vi "TCP Message Loop.vi"(8 "error in (no error)":errorcluster, 10 "Data Notifier":refnum<notifier>, 11 "Message Queues":T1) -> (0 "error out":errorcluster)   [LabVIEW 2026, in "TCP.lvlib"]
uses:
  TCP.lvlib
  Support/Message Queue/All Message Queues.ctl
  Support/Message Queue/Message Cluster.ctl
  Controls/Machine_State_Buffer.ctl
  Acquisition/Controls/Acquisition Metrics.ctl
  TCP State Data.ctl
  Controls/Telemetry_Data_Type.ctl
  Controls/Channels.ctl
  Support/Message Queue/Enqueue Message (Single).vi
  <vilib>/Utility/error.llb/Error Cluster From Error Code.vi
  <vilib>/ErrorRing/Error Ring.xnode
  support/Message Queue/Message Queue.lvlib
  Acquisition/Acquisition.lvlib
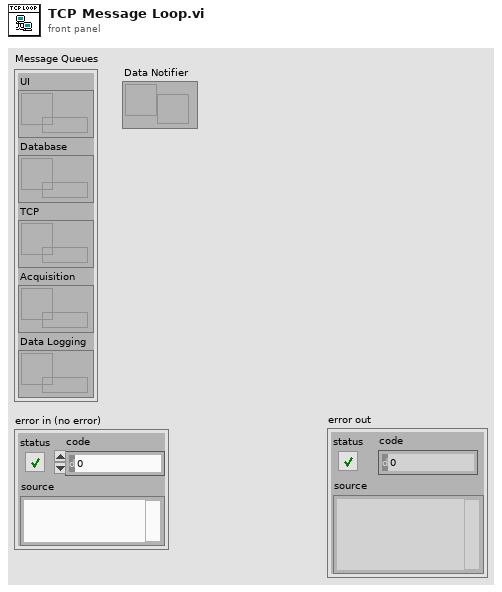
[diagram p1: front panel]
types:
  T1 = typedef "Message Queue.lvlib/All Message Queues.ctl" = cluster{"UI":refnum<queue>, "Database":refnum<queue>, "TCP":refnum<queue>, "Acquisition":refnum<queue>, "Data Logging":refnum<queue>}
  T2 = typedef "TCP.lvlib/TCP State Data.ctl" = cluster{"Connection ID":refnum<k5>, "Listener ID":refnum<k5>, "Is_Connected?":bool, "Last Time Check":dbl, "Error_Logged?":bool}
  T3 = typedef "Machine_State_Buffer.ctl" = cluster{"Waveforms":waveform(dbl)[], "Acquisition Metrics":T4}
  T4 = typedef "Acquisition.lvlib/Acquisition Metrics.ctl" = cluster{"Total_Samples":i64, "rpm":dbl}
  T5 = typedef "Telemetry_Data_Type.ctl" = cluster{"asset_id":i32, "frame_id":i32, "channels":T6, "comms/python link":bool, "rpm":dbl, "frequency_resolution":dbl}
  T6 = typedef "Channels.ctl" = cluster{"channel_id":dbl, "peak_frequency":dbl, "rms_acceleration":dbl, "health_score":dbl, "fft_magnitudes":dbl[]}[]
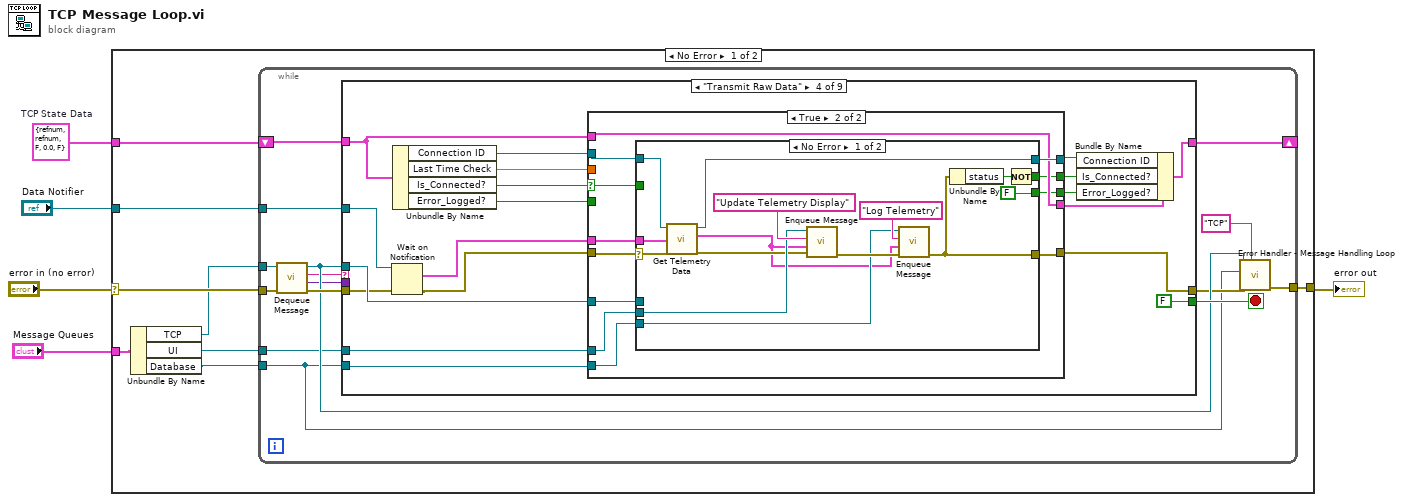
[diagram p0: block diagram]
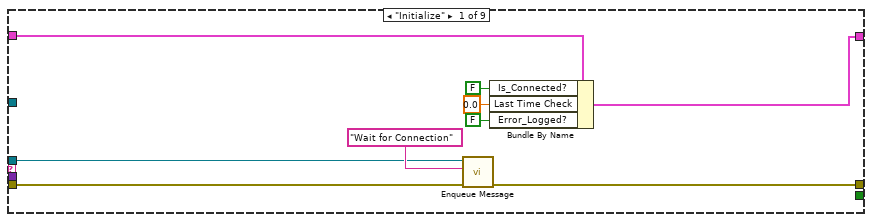
[diagram p2: hidden frame]
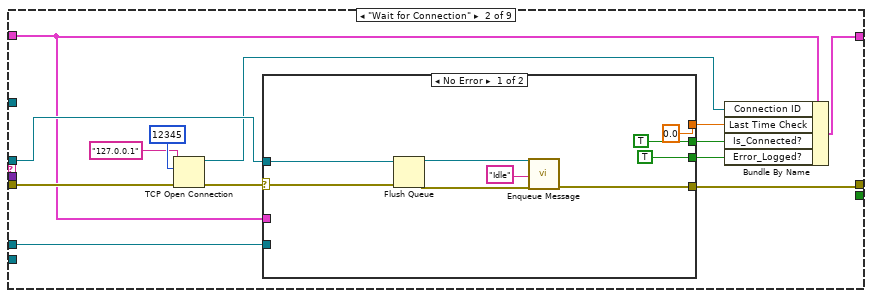
[diagram p3: hidden frame]
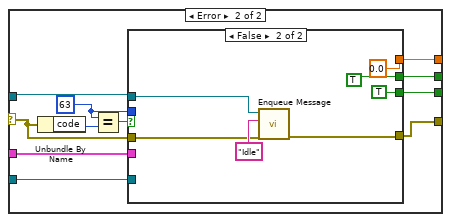
[diagram p4: hidden frame]
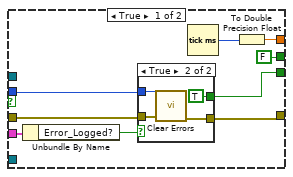
[diagram p5: hidden frame]
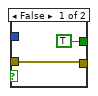
[diagram p6: hidden frame]
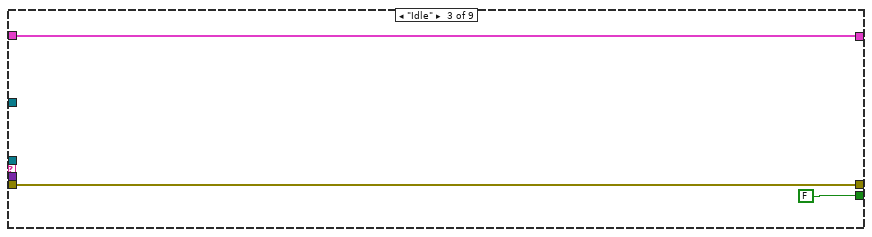
[diagram p7: hidden frame]
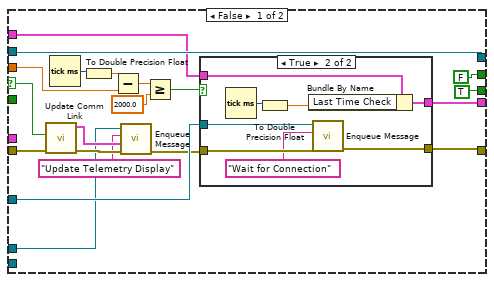
[diagram p8: hidden frame]
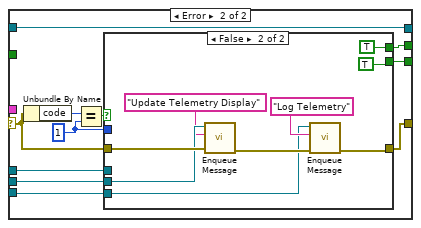
[diagram p10: hidden frame]
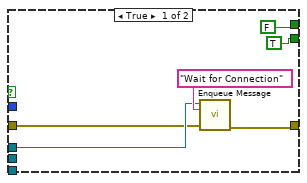
[diagram p11: hidden frame]
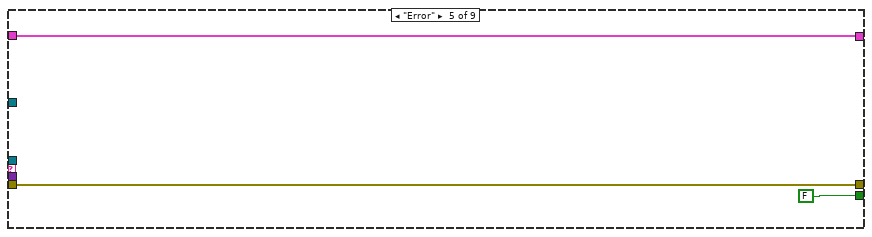
[diagram p12: hidden frame]
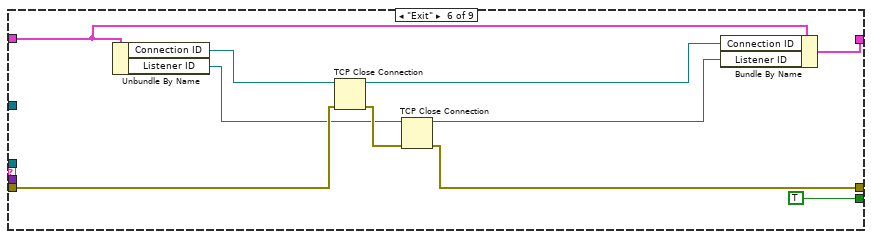
[diagram p13: hidden frame]
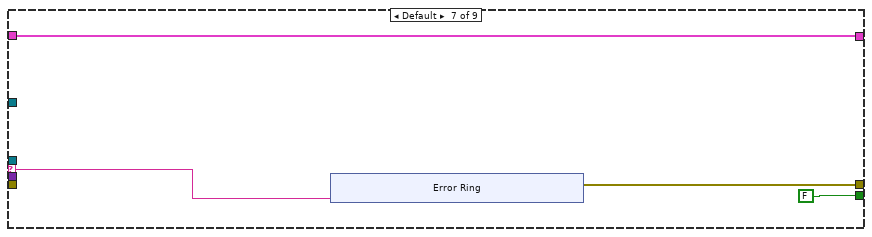
[diagram p14: hidden frame]
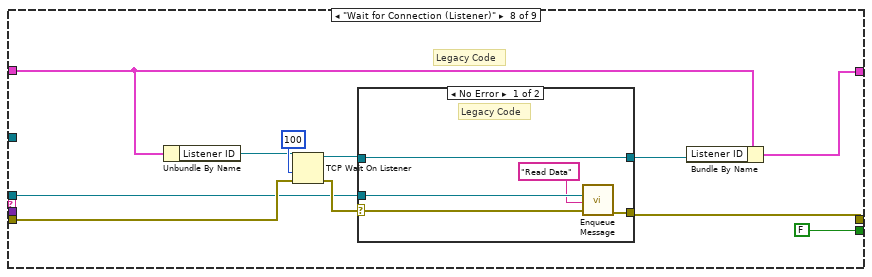
[diagram p15: hidden frame]
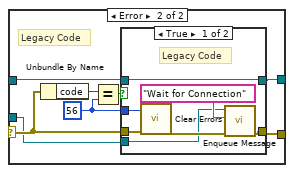
[diagram p16: hidden frame]
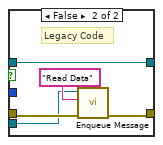
[diagram p17: hidden frame]
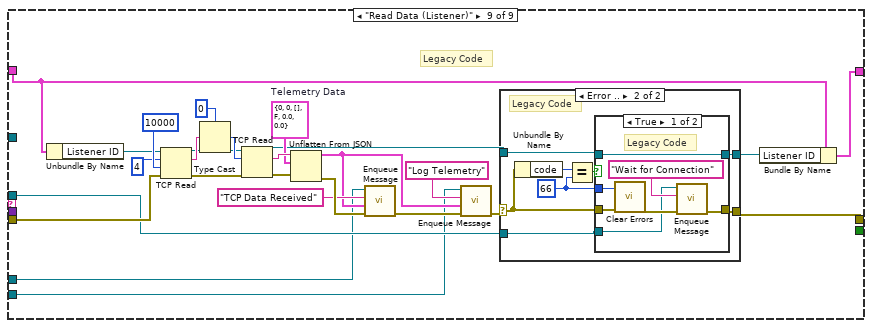
[diagram p18: hidden frame]
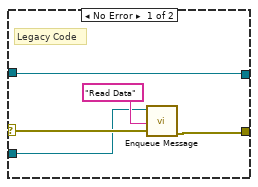
[diagram p19: hidden frame]
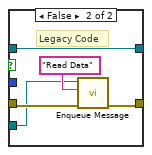
[diagram p20: hidden frame]
diagram:
  w2 = T2 {"Connection ID"=refnum, "Listener ID"=refnum, "Is_Connected?"=FALSE, "Last Time Check"=0.0, "Error_Logged?"=FALSE}  # TCP State Data
  n1 = case shown="No Error" "error in (no error)" {
    selector: "error in (no error)" -> [w12 w309]
    tunnel: [w13 w309] -> w5
    tunnel: "Message Queues" -> [w11 _]
    tunnel: w2 -> [w7 _]
    tunnel: "Data Notifier" -> [w6 _]
    frame No Error {
      n2 = Unbundle By Name(w11) -> ("TCP"=w10:refnum<queue>, "UI"=w8:refnum<queue>, "Database"=w9:refnum<queue>)
      n3 = while {
        tunnel: w12 -> [w28]
        tunnel: [w24] -> w13
        tunnel: w10 -> [w20]
        tunnel: w9 -> [w15]
        tunnel: w8 -> [w19]
        shift-right: [w17] -> _
        shift-left: w7 -> [w18]
        tunnel: w6 -> [w16]
        stop <- w26 stop-if-true
        n4 = call "Dequeue Message.vi"("error in (no error)"=w28, "Message Queue"=w20) -> ("error out"=w27:errorcluster, "Message Data"=w21:variant, "Message"=w22:string, "dup Message Queue"=w25:refnum<queue>)  [unwired: 6 in]
        n5 = case shown="\"Transmit Raw Data\"" w22 {
          selector: w22 -> [_ _ _ _ _ _ w213 _ _]
          tunnel: w25 -> [w36 w46 _ w108 _ _ _ w229 w269]
          tunnel: w27 -> [w35 w49 w94 w104 w199 w208 _ w230 w271]
          tunnel: [_ _ FALSE FALSE FALSE TRUE FALSE FALSE _] -> w26
          tunnel: [w29 w47 w94 w110 w199 w210 w212 w228 w283] -> w23
          tunnel: w21 -> [_ _ _ _ _ _ _ _ _]
          tunnel: w15 -> [_ _ _ w111 _ _ _ _ w262]
          tunnel: w19 -> [_ w38 _ w112 _ _ _ _ w263]
          tunnel: w18 -> [w34 w42 w93 w100 w198 w205 w211 w223 w260]
          tunnel: [w33 w45 w93 w109 w198 w203 w211 w222 w258] -> w17
          tunnel: w16 -> [_ _ _ w102 _ _ _ _ _]
          frame "Initialize" {
            n6 = call-poly "Enqueue Message.vi"("error in (no error)"=w35, "Message"="Wait for Connection", "Message Queue"=w36) -> ("error out"=w29:errorcluster)  [unwired: 7 in, 1 out]
            n7 = Bundle By Name(cluster=w34, "Is_Connected?"=FALSE, "Last Time Check"=0.0, "Error_Logged?"=FALSE) -> (w33:T2)
          }
          frame "Wait for Connection" {
            n8 = TCP Open Connection(address="127.0.0.1", remote port or service name=u16 12345, error in (no error)=w49) -> (connection ID=w40:refnum<k5>, error out=w39:errorcluster)  [unwired: 2 in]
            n9 = case shown="No Error" w39 {
              selector: w39 -> [w54 w69]
              tunnel: [w59 w66] -> w47
              tunnel: w46 -> [w52 w65]
              tunnel: [TRUE w64] -> w44
              tunnel: [0.0 w63] -> w43
              tunnel: w42 -> [_ w62]
              tunnel: [TRUE w61] -> w41
              tunnel: w38 -> [_ w60]
              frame No Error {
                n10 = Flush Queue(queue=w52, error in (no error)=w54) -> (queue out=w51:refnum<queue>, error out=w53:errorcluster)  [unwired: 1 out]
                n11 = call-poly "Enqueue Message.vi"("error in (no error)"=w53, "Message"="Idle", "Message Queue"=w51) -> ("error out"=w59:errorcluster)  [unwired: 7 in, 1 out]
              }
              frame Error {
                w68 = 63 ("y")
                n12 = Unbundle By Name(w69) -> ("code"=w67:i32)
                n13 = Equal?(x=w68, y=w67) -> (x = y?=w70:bool)
                n14 = case shown="False" w70 {
                  tunnel: w69 -> [w71 w86]
                  tunnel: [w76 w92] -> w66
                  tunnel: w68 -> [w72 _]
                  tunnel: w65 -> [_ w90]
                  tunnel: [FALSE TRUE] -> w64
                  tunnel: [w77 0.0] -> w63
                  tunnel: w62 -> [w75 _]
                  tunnel: [w73 TRUE] -> w61
                  tunnel: w60 -> [_ _]
                  frame True {
                    n15 = Unbundle By Name(w75) -> ("Error_Logged?"=w74:bool)
                    n16 = case shown="True" w74 {
                      tunnel: [w80 w85] -> w76
                      tunnel: w72 -> [_ w84]
                      tunnel: [TRUE TRUE] -> w73
                      tunnel: w71 -> [w80 w82]
                      frame False {
                      }
                      frame True {
                        n17 = call <vilib>:"Clear Errors.vi"("error in (no error)"=w82, "specific error code to clear (0: all)"=w84) -> ("error out"=w85:errorcluster)  [unwired: 4 in, 1 out]
                      }
                    }
                    n18 = Tick Count (ms)() -> (millisecond timer value=w78:u32)
                    n19 = To Double Precision Float(number=w78) -> (double precision float=w77:dbl)
                  }
                  frame False {
                    n20 = call-poly "Enqueue Message.vi"("error in (no error)"=w86, "Message"="Idle", "Message Queue"=w90) -> ("error out"=w92:errorcluster)  [unwired: 7 in, 1 out]
                  }
                }
              }
            }
            n21 = Bundle By Name(cluster=w42, "Connection ID"=w40, "Last Time Check"=w43, "Is_Connected?"=w44, "Error_Logged?"=w41) -> (w45:T2)
          }
          frame "Idle" {
          }
          frame "Transmit Raw Data" {
            n22 = Wait on Notification(notifier=w102, error in (no error)=w104) -> (notification=w101:T3, error out=w103:errorcluster)  [unwired: 2 in, 2 out]
            n23 = Unbundle By Name(w100) -> ("Connection ID"=w107:refnum<k5>, "Last Time Check"=w105:dbl, "Is_Connected?"=w113:bool, "Error_Logged?"=w98:bool)
            n24 = case shown="True" w113 {
              selector: w113 -> [w116 w145]
              tunnel: w103 -> [w118 w154]
              tunnel: w101 -> [_ w156]
              tunnel: [w134 w155] -> w110
              tunnel: w112 -> [w115 w153]
              tunnel: w111 -> [_ w152]
              tunnel: w108 -> [w133 w151]
              tunnel: w107 -> [w132 w150]
              tunnel: [w132 w149] -> w106
              tunnel: w105 -> [w129 _]
              tunnel: w100 -> [w126 w148]
              tunnel: [w125 w148] -> w99
              tunnel: w98 -> [_ _]
              tunnel: [FALSE w147] -> w97
              tunnel: [TRUE w146] -> w96
              frame False {
                n25 = call "Update Comm Link.vi"("error in (no error)"=w118, "Comms/Python Link"=w116) -> ("error out"=w120:errorcluster, "Telemetry Data out"=w121:T5)  [unwired: 8 in]
                n26 = Tick Count (ms)() -> (millisecond timer value=w131:u32)
                n27 = To Double Precision Float(number=w131) -> (double precision float=w130:dbl)
                n28 = Subtract(x=w130, y=w129) -> (x-y=w128:dbl)
                n29 = call-poly "Enqueue Message.vi"("error in (no error)"=w120, "Message Data"=w121, "Message"="Update Telemetry Display", "Message Queue"=w115) -> ("error out"=w117:errorcluster)  [unwired: 6 in, 1 out]
                n30 = Greater Or Equal?(x=w128, y=2000.0) -> (x >= y?=w122:bool)
                n31 = case shown="True" w122 {
                  tunnel: w117 -> [w136 w144]
                  tunnel: [w136 w143] -> w134
                  tunnel: w133 -> [_ w141]
                  tunnel: w126 -> [w135 w137]
                  tunnel: [w135 w138] -> w125
                  frame False {
                  }
                  frame True {
                    n32 = Tick Count (ms)() -> (millisecond timer value=w140:u32)
                    n33 = To Double Precision Float(number=w140) -> (double precision float=w139:dbl)
                    n34 = Bundle By Name(cluster=w137, "Last Time Check"=w139) -> (w138:T2)
                    n35 = call-poly "Enqueue Message.vi"("error in (no error)"=w144, "Message"="Wait for Connection", "Message Queue"=w141) -> ("error out"=w143:errorcluster)  [unwired: 7 in, 1 out]
                  }
                }
              }
              frame True {
                n36 = case shown="No Error" w154 {
                  selector: w154 -> [w165 w178]
                  tunnel: w156 -> [w171 _]
                  tunnel: [w162 w179] -> w155
                  tunnel: w153 -> [w167 w176]
                  tunnel: w152 -> [w166 w175]
                  tunnel: w151 -> [_ w177]
                  tunnel: w150 -> [w164 w174]
                  tunnel: [w163 w174] -> w149
                  tunnel: [w160 w173] -> w147
                  tunnel: [FALSE w172] -> w146
                  tunnel: w145 -> [_ _]
                  frame No Error {
                    n37 = call "Get Telemetry Data.vi"("error in (no error)"=w165, "Machine State Buffer"=w171, "TCP Network Connection in"=w164) -> ("error out"=w158:errorcluster, "Telemetry Data"=w157:T5, "TCP Network Connection out"=w163:refnum<k5>)  [unwired: 6 in]
                    n38 = call-poly "Enqueue Message.vi"("error in (no error)"=w158, "Message Data"=w157, "Message"="Update Telemetry Display", "Message Queue"=w167) -> ("error out"=w168:errorcluster)  [unwired: 6 in, 1 out]
                    n39 = call-poly "Enqueue Message.vi"("error in (no error)"=w168, "Message Data"=w157, "Message"="Log Telemetry", "Message Queue"=w166) -> ("error out"=w162:errorcluster)  [unwired: 6 in, 1 out]
                    n40 = Unbundle By Name(w162) -> ("status"=w161:bool)
                    n41 = Not(x=w161) -> (.not. x?=w160:bool)
                  }
                  frame Error {
                    w180 = 1 ("y")
                    n42 = Unbundle By Name(w178) -> ("code"=w182:i32)
                    n43 = Equal?(x=w182, y=w180) -> (x = y?=w181:bool)
                    n44 = case shown="False" w181 {
                      tunnel: w178 -> [w185 w195]
                      tunnel: [w188 w194] -> w179
                      tunnel: w180 -> [_ _]
                      tunnel: w177 -> [w186 _]
                      tunnel: w176 -> [_ w193]
                      tunnel: w175 -> [_ w192]
                      tunnel: [FALSE TRUE] -> w173
                      tunnel: [TRUE TRUE] -> w172
                      frame True {
                        n45 = call-poly "Enqueue Message.vi"("error in (no error)"=w185, "Message"="Wait for Connection", "Message Queue"=w186) -> ("error out"=w188:errorcluster)  [unwired: 7 in, 1 out]
                      }
                      frame False {
                        n46 = call-poly "Enqueue Message.vi"("error in (no error)"=w195, "Message"="Update Telemetry Display", "Message Queue"=w193) -> ("error out"=w197:errorcluster)  [unwired: 7 in, 1 out]
                        n47 = call-poly "Enqueue Message.vi"("error in (no error)"=w197, "Message"="Log Telemetry", "Message Queue"=w192) -> ("error out"=w194:errorcluster)  [unwired: 7 in, 1 out]
                      }
                    }
                  }
                }
              }
            }
            n48 = Bundle By Name(cluster=w99, "Connection ID"=w106, "Is_Connected?"=w97, "Error_Logged?"=w96) -> (w109:T2)
          }
          frame "Error" {
          }
          frame "Exit" {
            n49 = Unbundle By Name(w205) -> ("Connection ID"=w206:refnum<k5>, "Listener ID"=w202:refnum<k5>)
            n50 = TCP Close Connection(connection ID=w206, error in (no error)=w208) -> (connection ID out=w204:refnum<k5>, error out=w207:errorcluster)  [unwired: 1 in]
            n51 = TCP Close Connection(connection ID=w202, error in (no error)=w207) -> (connection ID out=w201:refnum<k5>, error out=w210:errorcluster)  [unwired: 1 in]
            n52 = Bundle By Name(cluster=w205, "Connection ID"=w204, "Listener ID"=w201) -> (w203:T2)
          }
          frame Default {
            n53 = xnode "Error Ring"("parameter 0"=w213) -> ("error out"=w212:errorcluster)
          }
          frame "Wait for Connection (Listener)" {
            # "Legacy Code"
            n54 = Unbundle By Name(w223) -> ("Listener ID"=w225:refnum<k5>)
            n55 = TCP Wait On Listener(8:w230, 9:100 ("timeout ms (wait forever: -1)"), 11:w225) -> (0:w231:errorcluster, 3:w226:refnum<k5>)  [unwired: 1 in, 3 out]
            n56 = case shown="No Error" w231 {
              selector: w231 -> [w234 w243]
              tunnel: w229 -> [w237 w240]
              tunnel: [w236 w242] -> w228
              tunnel: w226 -> [w233 w239]
              tunnel: [w233 w238] -> w224
              frame No Error {
                # "Legacy Code"
                n57 = call-poly "Enqueue Message.vi"("error in (no error)"=w234, "Message"="Read Data", "Message Queue"=w237) -> ("error out"=w236:errorcluster)  [unwired: 7 in, 1 out]
              }
              frame Error {
                w241 = 56 ("y")
                # "Legacy Code"
                n58 = Unbundle By Name(w243) -> ("code"=w245:i32)
                n59 = Equal?(x=w245, y=w241) -> (x = y?=w244:bool)
                n60 = case shown="True" w244 {
                  tunnel: w243 -> [w252 w255]
                  tunnel: [w250 w257] -> w242
                  tunnel: w241 -> [w248 _]
                  tunnel: w240 -> [w247 w254]
                  tunnel: w239 -> [w246 w253]
                  tunnel: [w246 w253] -> w238
                  frame True {
                    # "Legacy Code"
                    n61 = call <vilib>:"Clear Errors.vi"("error in (no error)"=w252, "specific error code to clear (0: all)"=w248) -> ("error out"=w251:errorcluster)  [unwired: 4 in, 1 out]
                    n62 = call-poly "Enqueue Message.vi"("error in (no error)"=w251, "Message"="Wait for Connection", "Message Queue"=w247) -> ("error out"=w250:errorcluster)  [unwired: 7 in, 1 out]
                  }
                  frame False {
                    # "Legacy Code"
                    n63 = call-poly "Enqueue Message.vi"("error in (no error)"=w255, "Message"="Read Data", "Message Queue"=w254) -> ("error out"=w257:errorcluster)  [unwired: 7 in, 1 out]
                  }
                }
              }
            }
            n64 = Bundle By Name(cluster=w223, "Listener ID"=w224) -> (w222:T2)
          }
          frame "Read Data (Listener)" {
            w275 = T5 {"asset_id"=0, "frame_id"=0, "channels"=[], "comms/python link"=FALSE, "rpm"=0.0, "frequency_resolution"=0.0}  # Telemetry Data
            # "Legacy Code"
            n65 = Unbundle By Name(w260) -> ("Listener ID"=w261:refnum<k5>)
            n66 = TCP Read(connection ID=w261, bytes to read=4, error in (no error)=w271, 9:10000 ("timeout ms (25000)")) -> (connection ID out=w270:refnum<k5>, data out=w277:string, error out=w280:errorcluster)  [unwired: 1 in]
            n67 = Type Cast(type=0, x=w277) -> (*(type *) &x=w278:i32)
            n68 = TCP Read(connection ID=w270, bytes to read=w278, error in (no error)=w280) -> (connection ID out=w268:refnum<k5>, data out=w279:string, error out=w281:errorcluster)  [unwired: 2 in]
            n69 = Unflatten From JSON(JSON string=w279, type and defaults=w275, error in (no error)=w281) -> (value=w265:T5, error out=w282:errorcluster)  [unwired: 4 in]
            n70 = call-poly "Enqueue Message.vi"("error in (no error)"=w282, "Message Data"=w265, "Message"="TCP Data Received", "Message Queue"=w263) -> ("error out"=w267:errorcluster)  [unwired: 6 in, 1 out]
            n71 = call-poly "Enqueue Message.vi"("error in (no error)"=w267, "Message Data"=w265, "Message"="Log Telemetry", "Message Queue"=w262) -> ("error out"=w266:errorcluster)  [unwired: 6 in, 1 out]
            n72 = case shown="Error .." w266 {
              selector: w266 -> [w286 w294]
              tunnel: [w288 w293] -> w283
              tunnel: w268 -> [w285 w291]
              tunnel: [w285 w290] -> w259
              tunnel: w269 -> [w284 w289]
              frame No Error {
                # "Legacy Code"
                n73 = call-poly "Enqueue Message.vi"("error in (no error)"=w286, "Message"="Read Data", "Message Queue"=w284) -> ("error out"=w288:errorcluster)  [unwired: 7 in, 1 out]
              }
              frame Error {
                w292 = 66 ("y")
                # "Legacy Code"
                n74 = Unbundle By Name(w294) -> ("code"=w296:i32)
                n75 = Equal?(x=w296, y=w292) -> (x = y?=w295:bool)
                n76 = case shown="True" w295 {
                  tunnel: w294 -> [w303 w306]
                  tunnel: [w301 w308] -> w293
                  tunnel: w292 -> [w299 _]
                  tunnel: w289 -> [w298 w305]
                  tunnel: w291 -> [w297 w304]
                  tunnel: [w297 w304] -> w290
                  frame True {
                    # "Legacy Code"
                    n77 = call <vilib>:"Clear Errors.vi"("error in (no error)"=w303, "specific error code to clear (0: all)"=w299) -> ("error out"=w302:errorcluster)  [unwired: 4 in, 1 out]
                    n78 = call-poly "Enqueue Message.vi"("error in (no error)"=w302, "Message"="Wait for Connection", "Message Queue"=w298) -> ("error out"=w301:errorcluster)  [unwired: 7 in, 1 out]
                  }
                  frame False {
                    # "Legacy Code"
                    n79 = call-poly "Enqueue Message.vi"("error in (no error)"=w306, "Message"="Read Data", "Message Queue"=w305) -> ("error out"=w308:errorcluster)  [unwired: 7 in, 1 out]
                  }
                }
              }
            }
            n80 = Bundle By Name(cluster=w260, "Listener ID"=w259) -> (w258:T2)
          }
        }
        n81 = call "Error Handler - Message Handling Loop.vi"("Loop Name"="TCP", "error in (no error)"=w23, "Database"=w15, "Message Queue"=w25) -> ("dup error in"=w24:errorcluster)  [unwired: 6 in, 1 out]
      }
    }
    frame Error {
    }
  }
  "error out" <- w5
